vi "CmdCenter_RFmx_Test.vi"(8 "error in (no error)":errorcluster, 11 "Message_Queues":T4) -> (0 "error out":errorcluster)   [LabVIEW 2014]
uses:
  15_DataManagement/Config_RFSG.ctl
  02_Controls/Message_Queues.ctl
  02_Controls/Message_Data_Ctl.ctl
  15_DataManagement/Config_RFmx_Settings.ctl
  15_DataManagement/RFmx_Analysis_Parameter.ctl
panel:
  in  "RFmx_An_Data":T1={"Center_Freq(Hz)"=1000000000.0, "Span(Hz)"=30000000.0, "Ch_IBW(Hz)"=3840000.0, "IMD_Tone_Spacing(Hz)"=3000000.0, "IMD_Span(Hz)"=30000000.0, "IMD_Ch_IBW(Hz)"=1000000.0, "IMD_TargPwr(dBm)"=-10.0, "SFDR_Span(Hz)"=50000000.0, "SFDR_Ch_IBW(Hz)"=2000000.0, "ACP_Offset_Freq"=[10000000.0, 7500000.0, 12500000.0], "ACP_Offset_IBW"=[9000000.0, 3840000.0, 3840000.0], "Display ?"=TRUE} {"ACP_Offset_IBW" format="%#_6p"; "ACP_Offset_Freq" format="%#_6p"; "SFDR_Ch_IBW(Hz)" format="%.3p"; "SFDR_Span(Hz)" format="%.3p"; "IMD_TargPwr(dBm)" format="%.3p"; "IMD_Ch_IBW(Hz)" format="%.3p"; "IMD_Span(Hz)" format="%.3p"; "IMD_Tone_Spacing(Hz)" format="%.3p"; "Ch_IBW(Hz)" format="%.3p"; "Span(Hz)" format="%.3p"; "Center_Freq(Hz)" format="%.3p"}
  in  "DispOn":bool
  in  "Fetch_Types":string[](array[string])=["Spectrum_Disp", "ACP_Data", "CHP_Data", "OBW_Data", "TXP_Data", "TXP_Disp", "CCDF_Data", "CCDF_Disp", "Harmonics_Disp"]
  in  "Meas_Types":string[](array[string])=["Spectrum", "ACP", "CHP", "OBW", "TXP", "CCDF", "Harmonics"]
  in  "RFmx_Parameters":T2={"Default"={"Center_Freq(Hz)"=1000000000.0, "Ref_Level(dBm)"=-5.0, "Span(Hz)"=30000000.0, "RBW(Hz)"=10000.0, "RBW Filter Type"=enum."Gaussian", "Ch_IBW(Hz)"=3840000.0, "Sweep_Time(s)"=0.01, "Num_of_Average"=10, "IQ_Bandwidth(Hz)"=20000000.0}, "ACP_Offset_Freq"=[10000000.0, 7500000.0, 12500000.0], "ACP_Offset_IBW"=[9000000.0, 3840000.0, 3840000.0], "OBW_Percent(%)"=95.0, "TXP_Interval(s)"=0.01, "CCDF_Interval(s)"=0.01, "CCDF_Threshold"=-30.0, "SFDR_Span(Hz)"=20000000.0, "Harms_RBW(Hz)"=100000.0, "Harms_RBW_Filter"=enum."Gaussian"} {"Harms_RBW(Hz)" format="%.3p"; "TXP_Interval(s)" format="%#_6p"; "SFDR_Span(Hz)" format="%#_6p"; "CCDF_Threshold" format="%#_6p"; "CCDF_Interval(s)" format="%#_6p"; "OBW_Percent(%)" format="%#_6p"; "ACP_Offset_IBW" format="%#_6p"; "ACP_Offset_Freq" format="%#_6p"; "Default"."IQ_Bandwidth(Hz)" format="%#_6p"; "Default"."Sweep_Time(s)" format="%#_6p"; "Default"."Ch_IBW(Hz)" format="%.3p"; "Default"."RBW(Hz)" format="%.3p"; "Default"."Span(Hz)" format="%.3p"; "Default"."Ref_Level(dBm)" format="%.3p"; "Default"."Center_Freq(Hz)" format="%.3p"}
  in  "Config_RFSG":T3={"Carrier Frequency"=1000000000.0, "RF Power Level (dBm)"=-10.0, "SG External Gain (dBm)"=0.0, "Standard"=enum."WCDMA"} {"SG External Gain (dBm)" format="%#_6p"; "RF Power Level (dBm)" format="%#_6p"; "Carrier Frequency" format="%#_6p"}
  out "Current_Message":string="OK"
  in  "Stop Button":bool
  in  "Start":bool
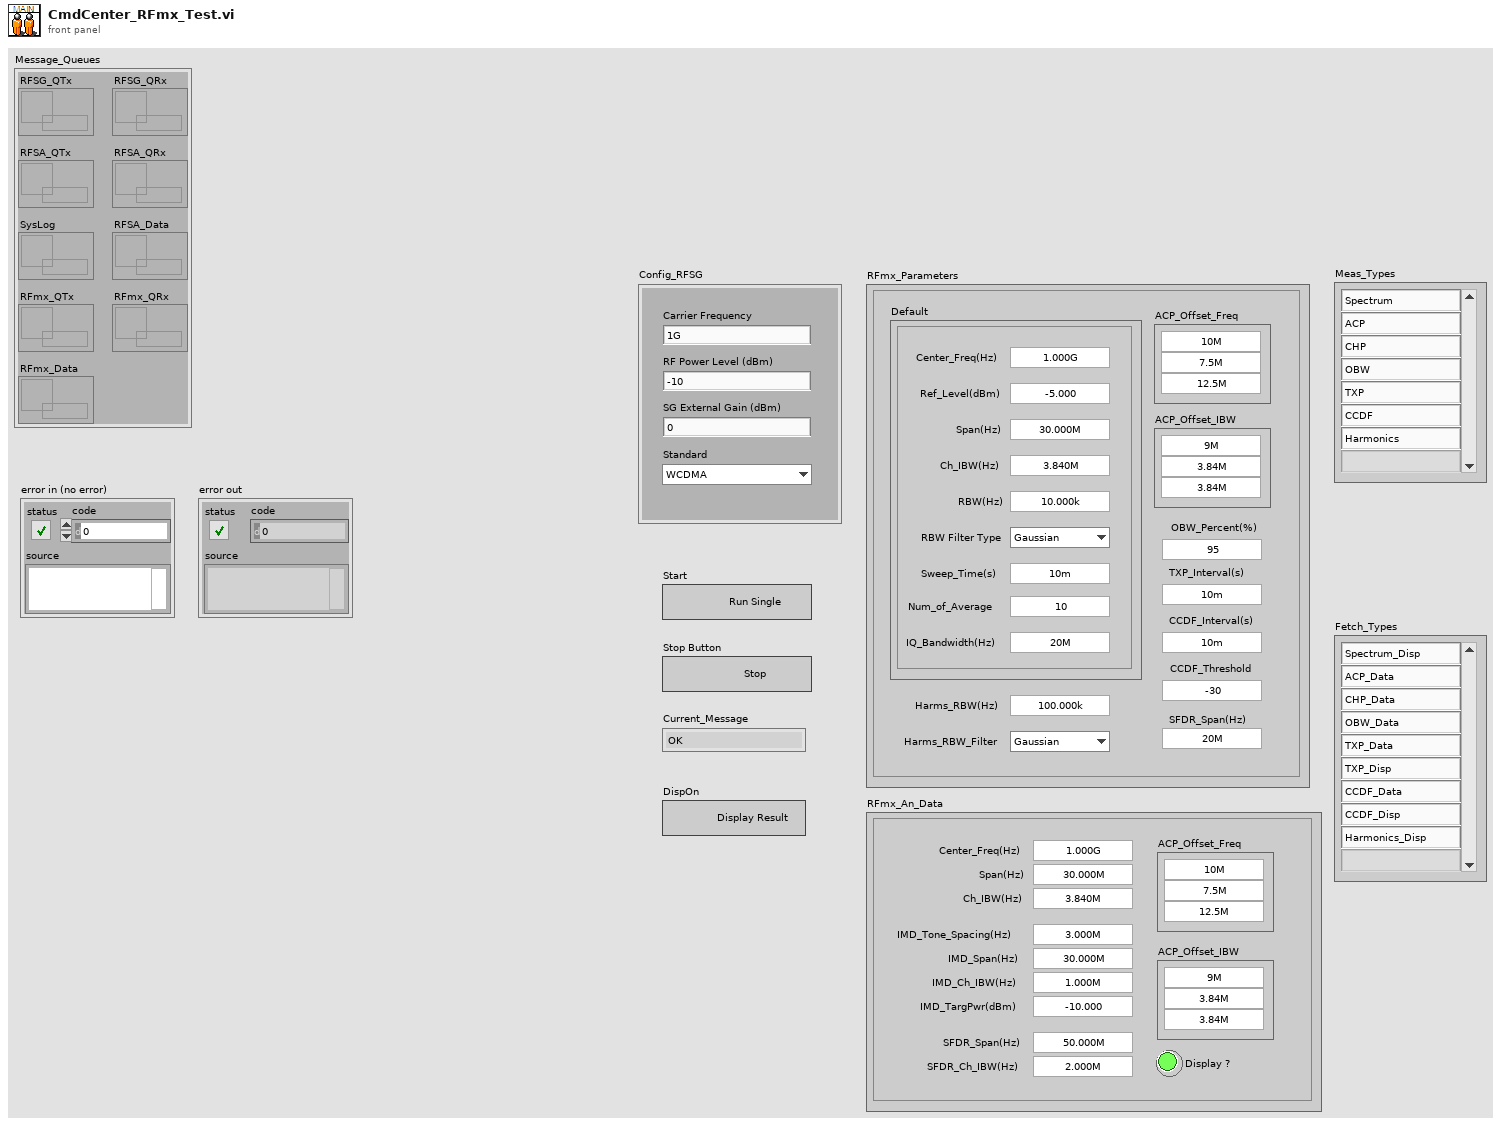
[diagram p1: front panel]
types:
  T1 = typedef "RFmx_Analysis_Parameter.ctl" = cluster{"Center_Freq(Hz)":dbl, "Span(Hz)":dbl, "Ch_IBW(Hz)":dbl, "IMD_Tone_Spacing(Hz)":dbl, "IMD_Span(Hz)":dbl, "IMD_Ch_IBW(Hz)":dbl, "IMD_TargPwr(dBm)":dbl, "SFDR_Span(Hz)":dbl, "SFDR_Ch_IBW(Hz)":dbl, "ACP_Offset_Freq":dbl[], "ACP_Offset_IBW":dbl[], "Display ?":bool}
  T2 = typedef "Config_RFmx_Settings.ctl" = cluster{"Default":cluster{"Center_Freq(Hz)":dbl, "Ref_Level(dBm)":dbl, "Span(Hz)":dbl, "RBW(Hz)":dbl, "RBW Filter Type":enum16{"FFT Based", "Gaussian", "Flat", "Synch Tuned - 4", "Synch Tuned - 5"}, "Ch_IBW(Hz)":dbl, "Sweep_Time(s)":dbl, "Num_of_Average":i32, "IQ_Bandwidth(Hz)":dbl}, "ACP_Offset_Freq":dbl[], "ACP_Offset_IBW":dbl[], "OBW_Percent(%)":dbl, "TXP_Interval(s)":dbl, "CCDF_Interval(s)":dbl, "CCDF_Threshold":dbl, "SFDR_Span(Hz)":dbl, "Harms_RBW(Hz)":dbl, "Harms_RBW_Filter":enum16{"FFT Based", "Gaussian", "Flat", "Synch Tuned - 4", "Synch Tuned - 5"}}
  T3 = typedef "Config_RFSG.ctl" = cluster{"Carrier Frequency":dbl, "RF Power Level (dBm)":dbl, "SG External Gain (dBm)":dbl, "Standard":enum16{"LTE", "WCDMA", "GSM", "EDGE", "CW", "CWM"}}
  T4 = typedef "Message_Queues.ctl" = cluster{"RFSG_QTx":refnum<queue>, "RFSG_QRx":refnum<queue>, "RFSA_QTx":refnum<queue>, "RFSA_QRx":refnum<queue>, "SysLog":refnum<queue>, "RFSA_Data":refnum<queue>, "RFmx_QTx":refnum<queue>, "RFmx_QRx":refnum<queue>, "RFmx_Data":refnum<queue>}
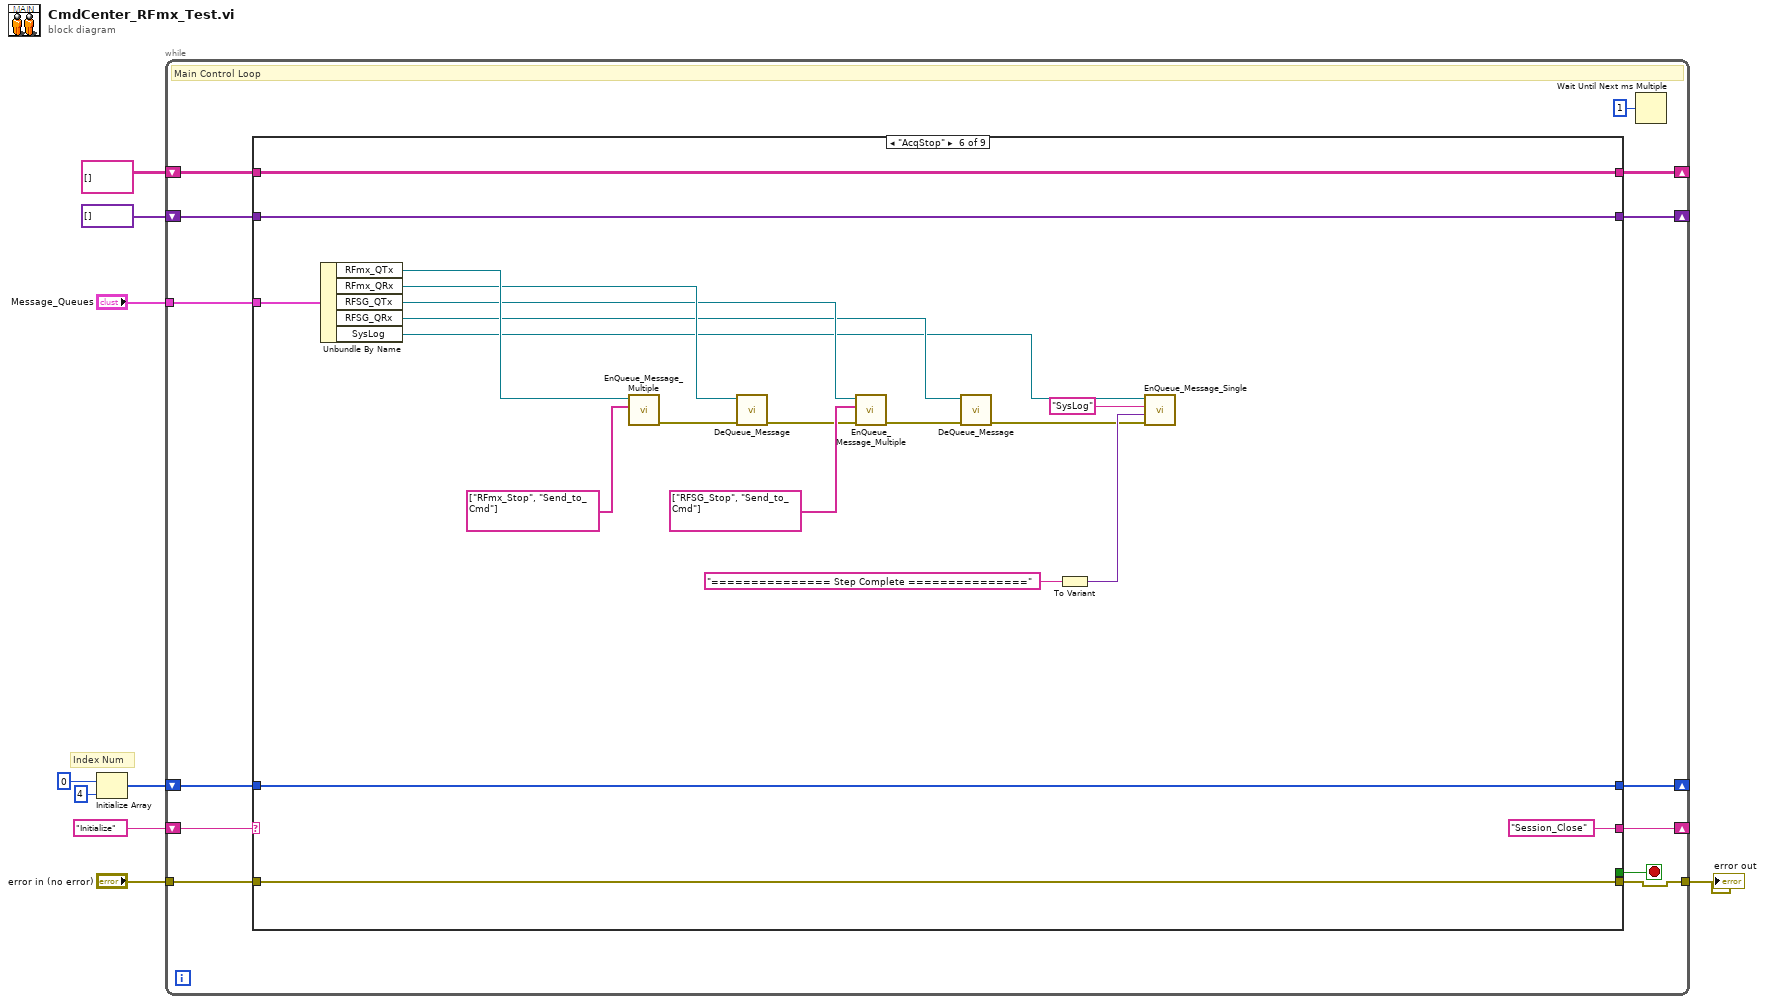
[diagram p0: block diagram]
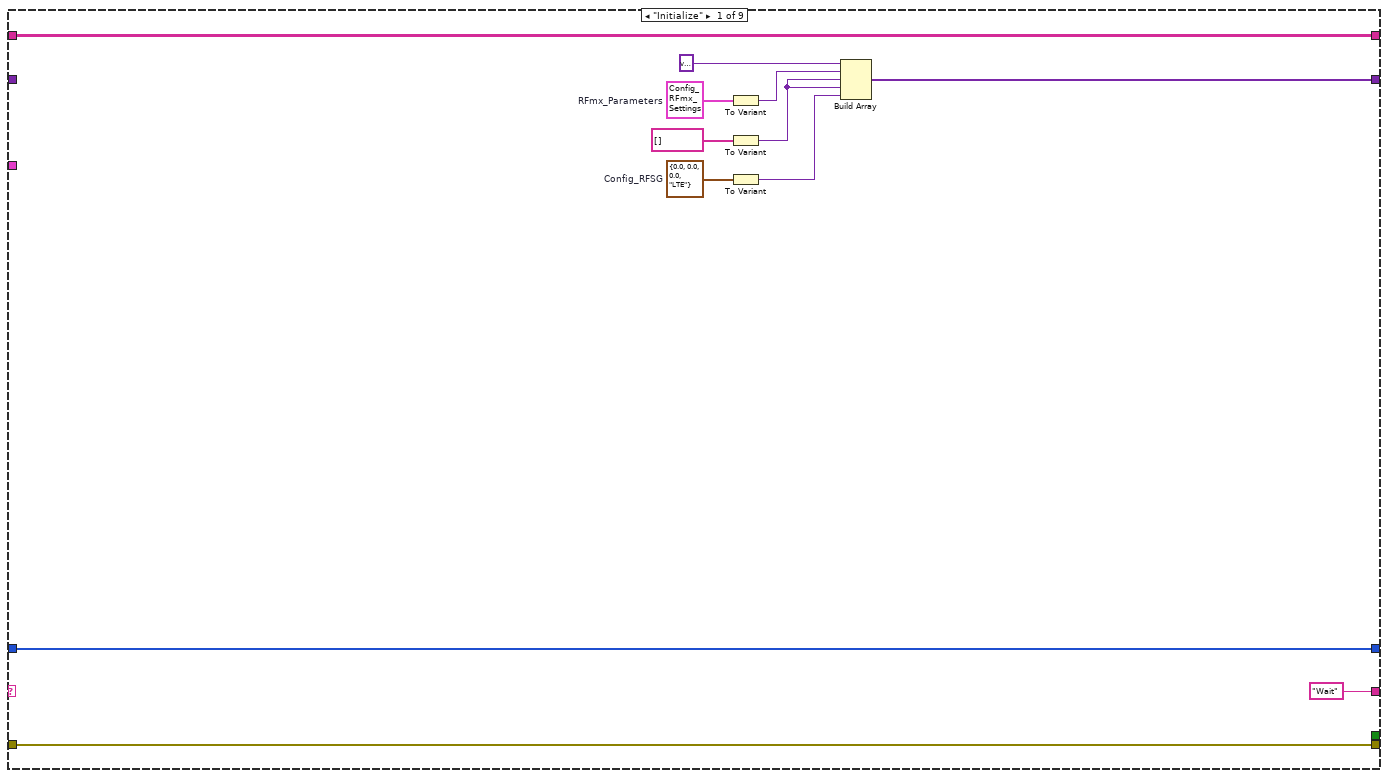
[diagram p2: hidden frame]
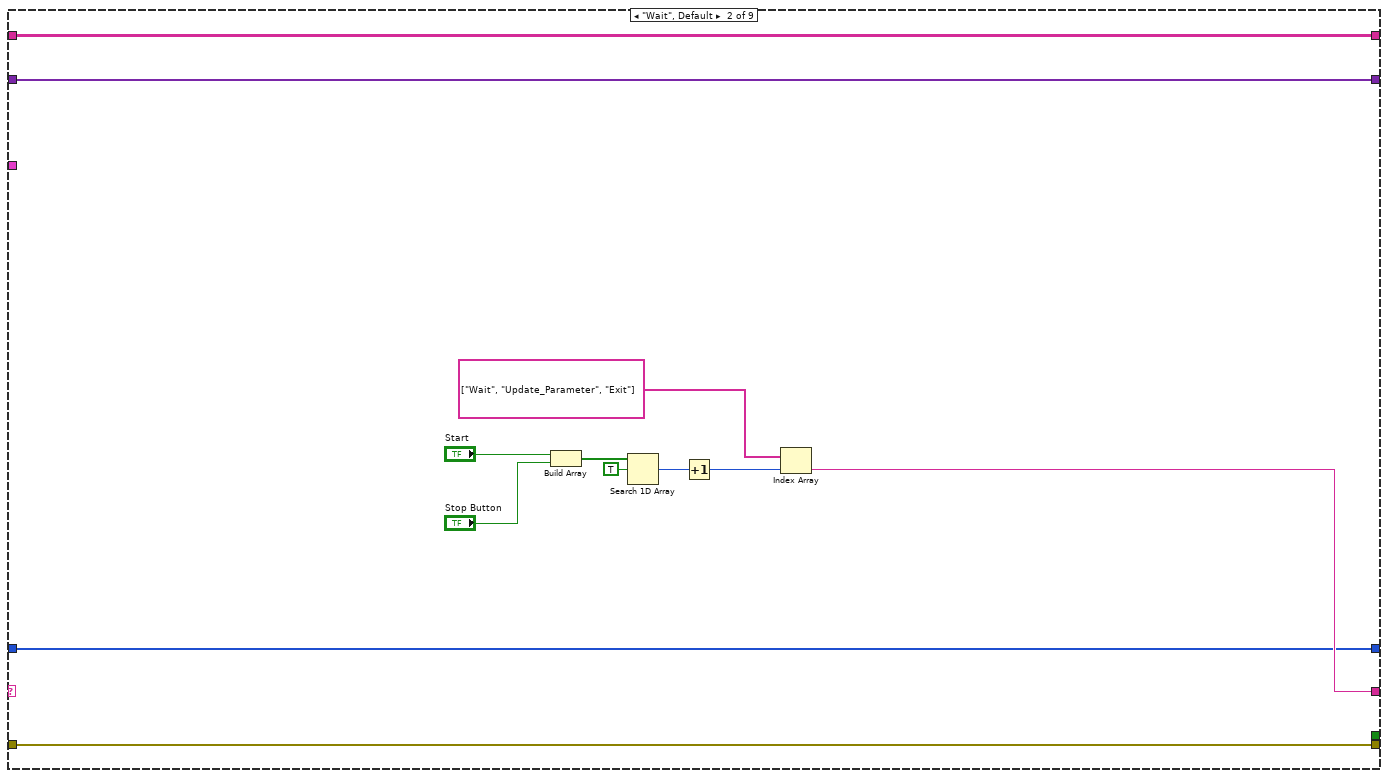
[diagram p3: hidden frame]
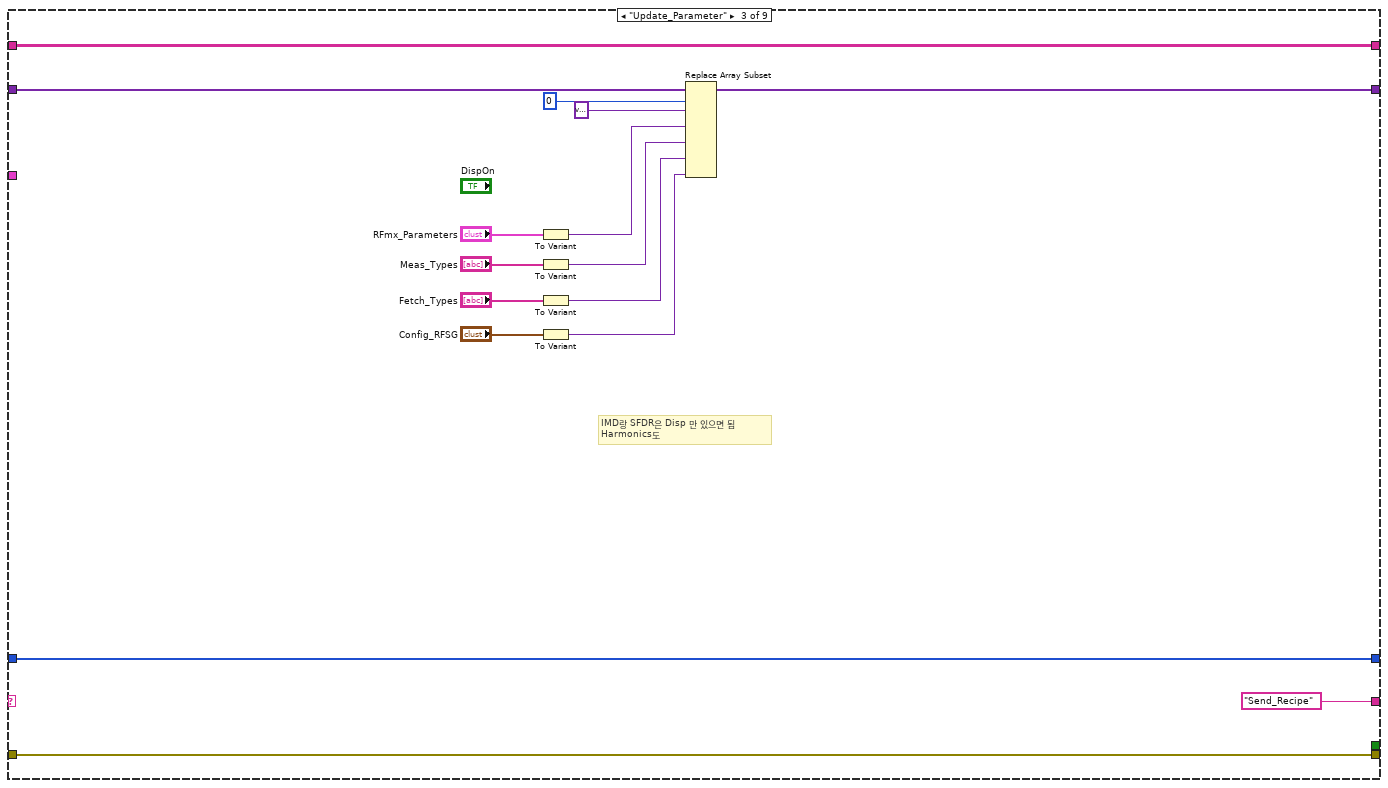
[diagram p4: hidden frame]
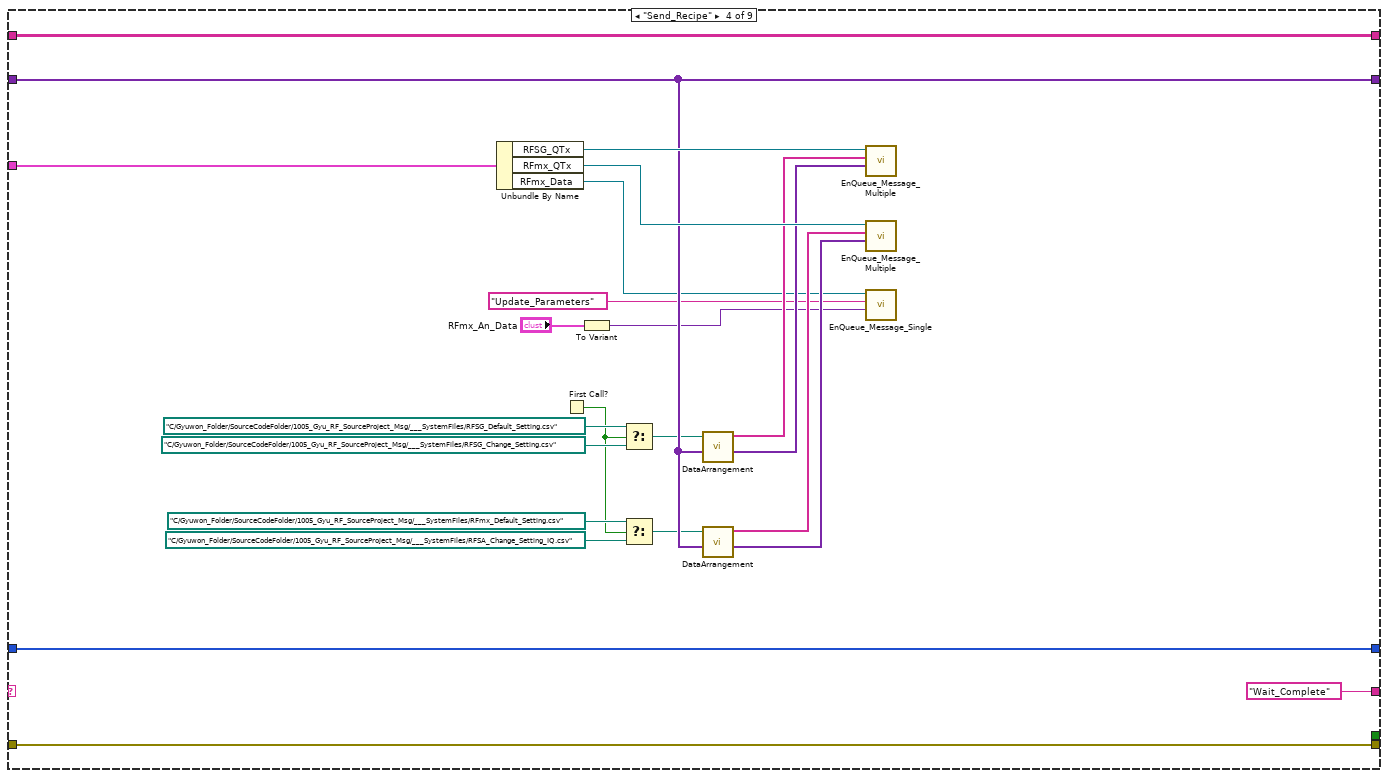
[diagram p5: hidden frame]
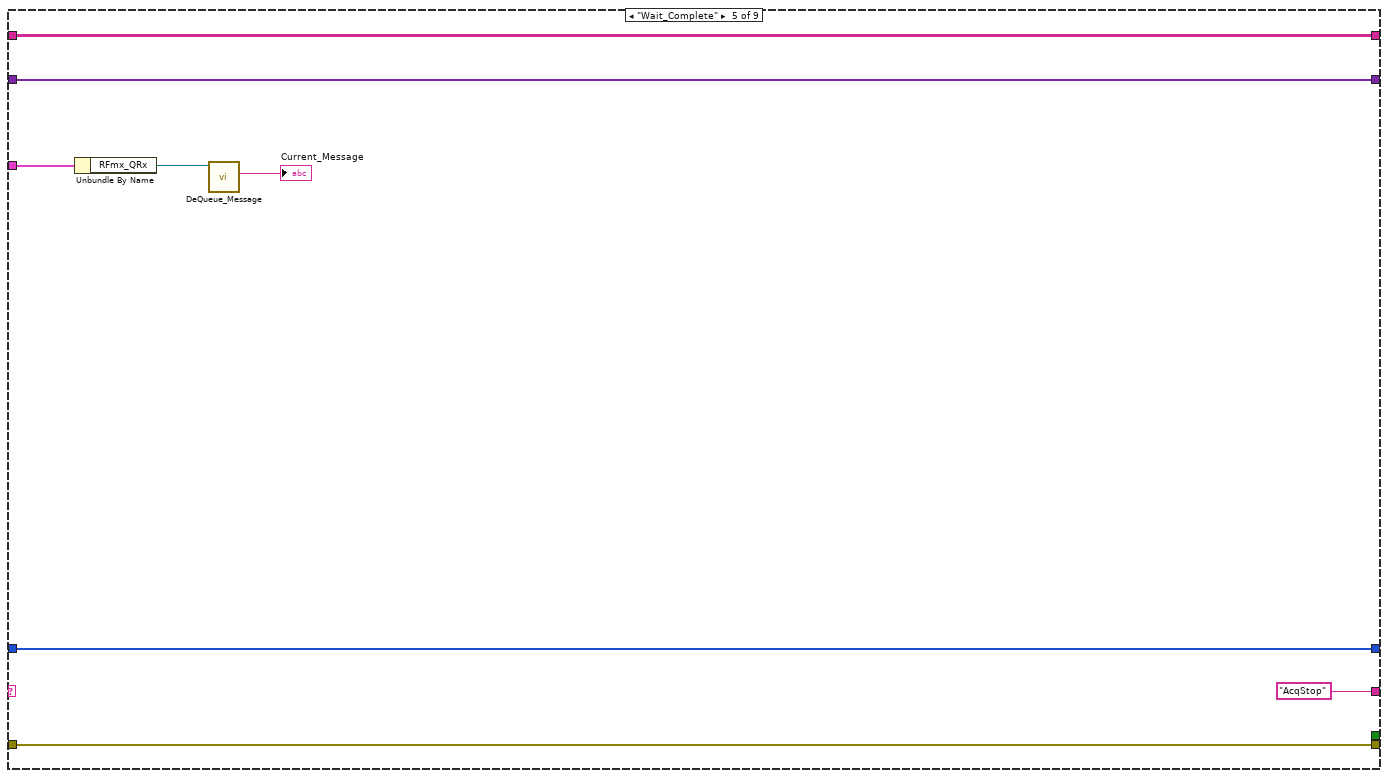
[diagram p6: hidden frame]
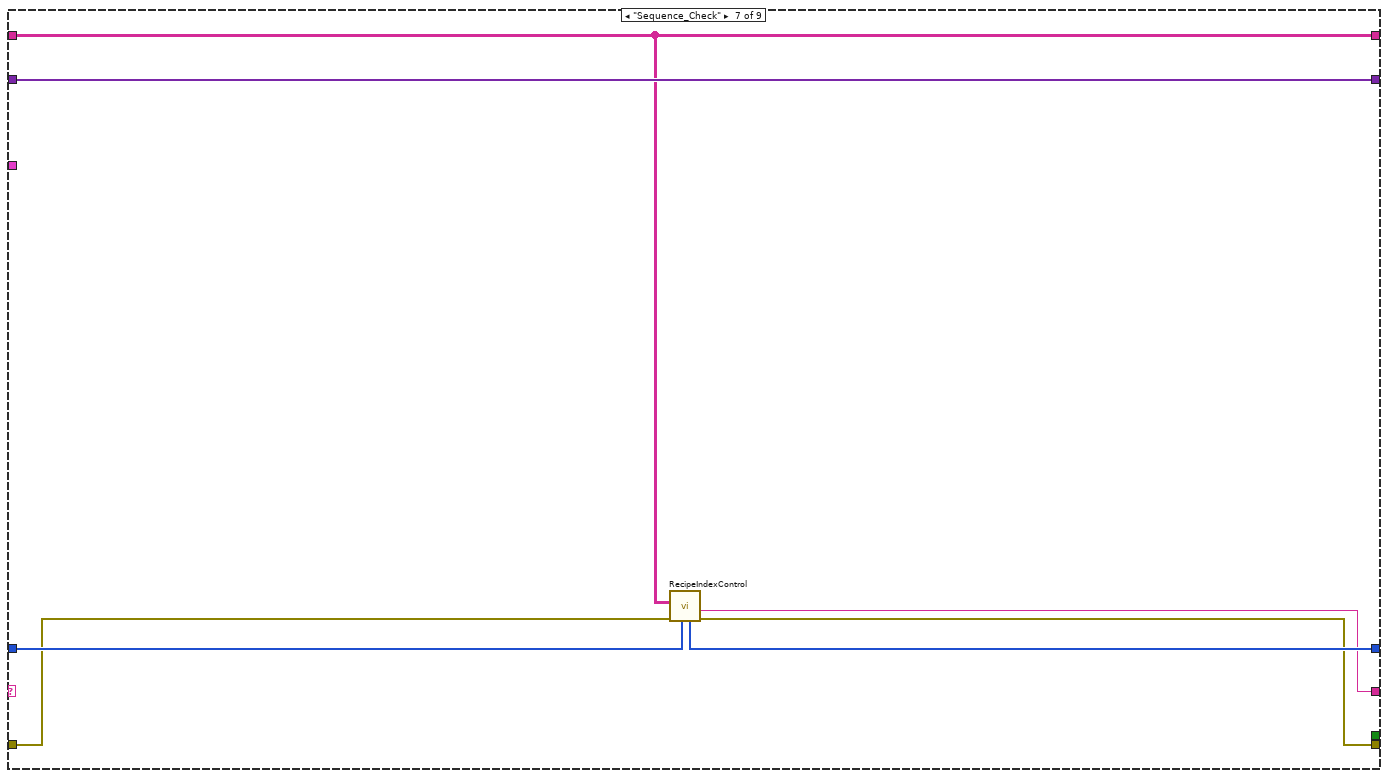
[diagram p7: hidden frame]
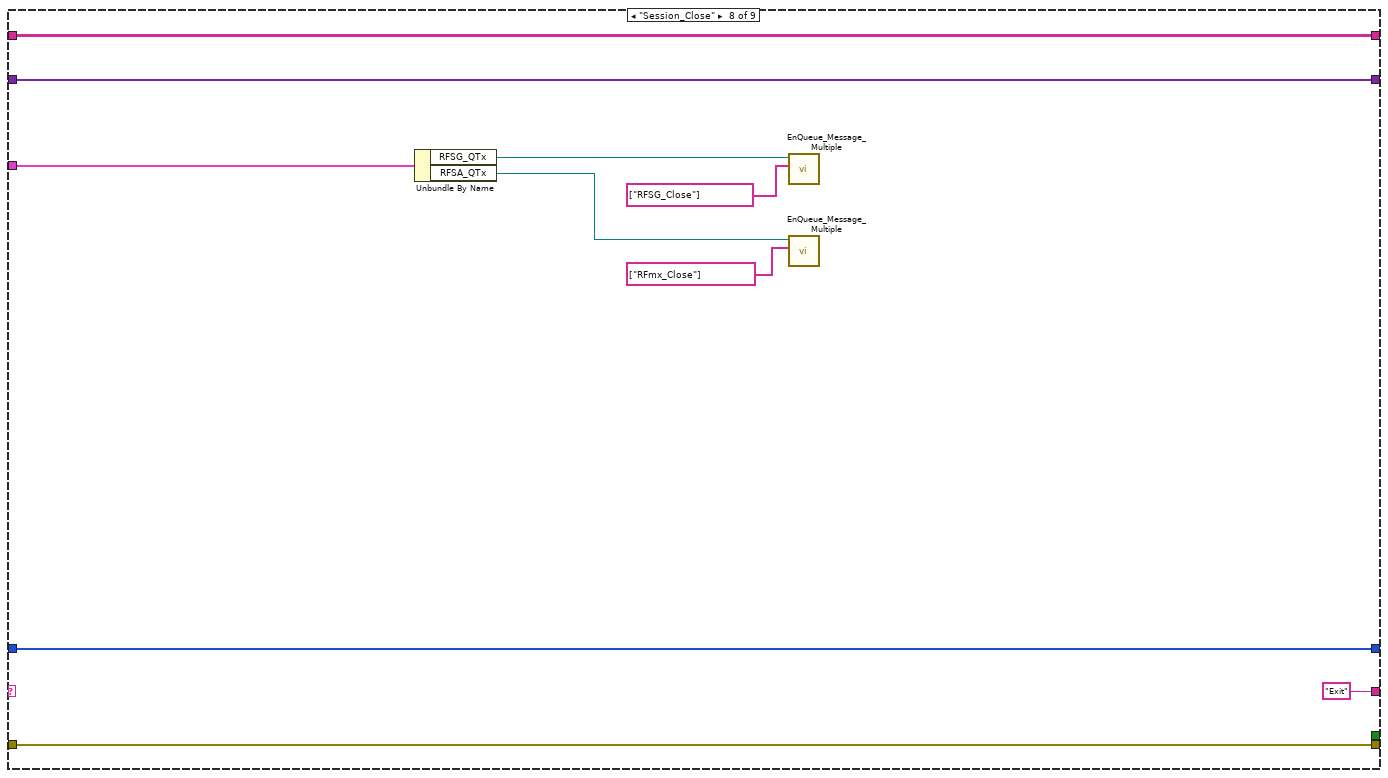
[diagram p8: hidden frame]
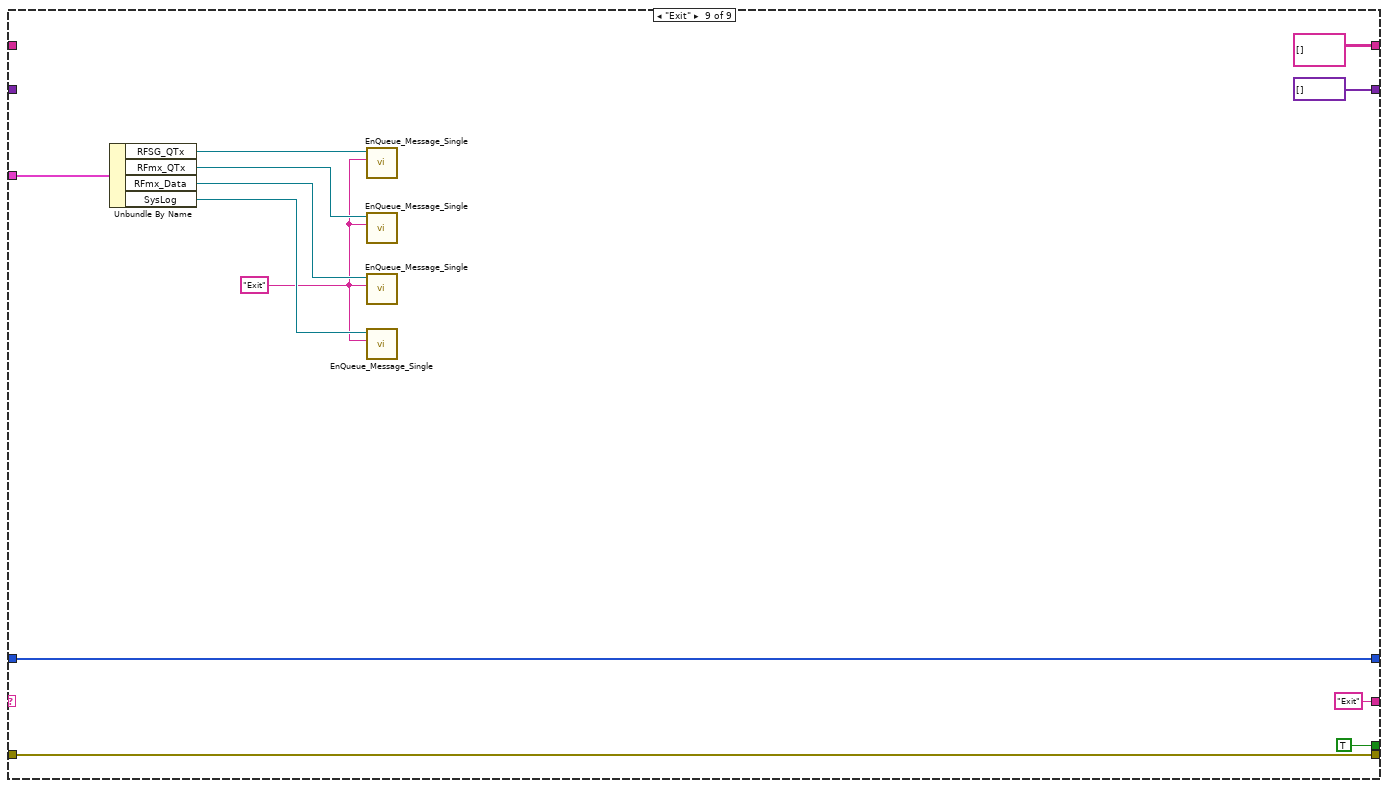
[diagram p9: hidden frame]
diagram:
  # "Index Num"
  n1 = Initialize Array(0, 4 ("dimension size")) -> (w1:i32[])
  n2 = while {
    tunnel: "error in (no error)" -> [w18]
    tunnel: [w21] -> w8
    tunnel: "Message_Queues" -> [w19]
    shift-right: [w16] -> _
    shift-left: "Initialize" -> [w20]
    shift-right: [w14] -> _
    shift-left: variant[] [] ("appended array") -> [w15]
    shift-right: [w13] -> _
    shift-left: string[][] [] ("all rows") -> [w12]
    shift-right: [w10] -> _
    shift-left: w1 -> [w11]
    stop <- w22 stop-if-true
    # "Main Control Loop"
    n3 = case shown="\"AcqStop\"" w20 {
      tunnel: w18 -> [w34 w46 w53 w85 w93 w110 w117 w124 w141]
      tunnel: [_ _ _ _ _ _ _ _ TRUE] -> w22
      tunnel: [w34 w46 w53 w85 w93 w110 w114 w124 w141] -> w21
      tunnel: w19 -> [_ _ _ w84 w91 w112 _ w129 w139]
      tunnel: ["Wait" w40 "Send_Recipe" "Wait_Complete" "AcqStop" "Session_Close" w116 "Exit" "Exit"] -> w16
      tunnel: w15 -> [_ w39 w59 w76 w88 w109 w120 w123 _]
      tunnel: [w31 w39 w58 w76 w88 w109 w120 w123 variant[] [] ("appended array")] -> w14
      tunnel: [w30 w38 w61 w75 w87 w108 w115 w122 string[][] [] ("all rows")] -> w13
      tunnel: w12 -> [w30 w38 w61 w75 w87 w108 w115 w122 _]
      tunnel: w11 -> [w29 w37 w60 w74 w86 w107 w119 w121 w131]
      tunnel: [w29 w37 w60 w74 w86 w107 w118 w121 w131] -> w10
      frame "Initialize" {
        w28 = T2 {"Default"={"Center_Freq(Hz)"=1150000000.0, "Ref_Level(dBm)"=-10.0, "Span(Hz)"=20000000.0, "RBW(Hz)"=10000.0, "RBW Filter Type"=enum."Gaussian", "Ch_IBW(Hz)"=3840000.0, "Sweep_Time(s)"=0.01, "Num_of_Average"=10, "IQ_Bandwidth(Hz)"=20000000.0}, "ACP_Offset_Freq"=[5000000.0, 10000000.0, 12500000.0], "ACP_Offset_IBW"=[3840000.0, 3840000.0, 3840000.0], "OBW_Percent(%)"=95.0, "TXP_Interval(s)"=0.01, "CCDF_Interval(s)"=0.01, "CCDF_Threshold"=-30.0, "SFDR_Span(Hz)"=20000000.0, "Harms_RBW(Hz)"=10000.0, "Harms_RBW_Filter"=enum."Gaussian"}  # RFmx_Parameters
        w32 = T3 {"Carrier Frequency"=0.0, "RF Power Level (dBm)"=0.0, "SG External Gain (dBm)"=0.0, "Standard"=enum."LTE"}  # Config_RFSG
        n4 = To Variant(anything=w28) -> (Variant=w27:variant)
        n5 = To Variant(anything=string[] []) -> (Variant=w23:variant)
        n6 = To Variant(anything=w32) -> (Variant=w26:variant)
        n7 = Build Array(variant ("element"), w27, w23, w23, w26) -> (w31:variant[])
      }
      frame "Wait", Default {
        n8 = Build Array("Start", "Stop Button") -> (w44:bool[])
        n9 = Search 1D Array(1D array=w44, element=TRUE) -> (index of element=w42:i32)  [unwired: 1 in]
        n10 = Increment(x=w42) -> (x+1=w41:i32)
        n11 = Index Array(array=string[] ["Wait", "Update_Parameter", "Exit"], index=w41) -> (element=w40:string)
      }
      frame "Update_Parameter" {
        # "IMD랑 SFDR은 Disp 만 있으면 됨\nHarmonics도"
        n12 = To Variant(anything="RFmx_Parameters") -> (Variant=w54:variant)
        n13 = To Variant(anything="Meas_Types") -> (Variant=w51:variant)
        n14 = To Variant(anything="Fetch_Types") -> (Variant=w47:variant)
        n15 = To Variant(anything="Config_RFSG") -> (Variant=w49:variant)
        n16 = Replace Array Subset(array=w59, new element #1=variant ("new element/subarray"), index #1=0 ("index"), new element #2=w54, new element #3=w51, new element #4=w47, new element #5=w49) -> (w58:variant[])  [unwired: 4 in]
      }
      frame "Send_Recipe" {
        n17 = Unbundle By Name(w84) -> ("RFSG_QTx"=w83:refnum<queue>, "RFmx_QTx"=w82:refnum<queue>, "RFmx_Data"=w66:refnum<queue>)
        n18 = First Call?() -> (First Call?: T/F=w69:bool)
        n19 = To Variant(anything="RFmx_An_Data") -> (Variant=w64:variant)
        n20 = Select(t=path "C:/Gyuwon_Folder/SourceCodeFolder/1005_Gyu_RF_SourceProject_Msg/___SystemFiles/RFSG_Default_Setting.csv" ("RFSG_List_1st"), s=w69, f=path "C:/Gyuwon_Folder/SourceCodeFolder/1005_Gyu_RF_SourceProject_Msg/___SystemFiles/RFSG_Change_Setting.csv" ("RFSG_List_1st")) -> (s? t:f=w68:path)
        n21 = Select(t=path "C:/Gyuwon_Folder/SourceCodeFolder/1005_Gyu_RF_SourceProject_Msg/___SystemFiles/RFmx_Default_Setting.csv" ("RFSA_List_1st"), s=w69, f=path "C:/Gyuwon_Folder/SourceCodeFolder/1005_Gyu_RF_SourceProject_Msg/___SystemFiles/RFSA_Change_Setting_IQ.csv" ("RFSA_List_1st")) -> (s? t:f=w67:path)
        n22 = call "DataArrangement.vi"("DataType"=w76, "file path (dialog if empty)"=w68) -> ("DataList"=w79:variant[], "CmdList"=w80:string[])  [unwired: 7 in, 1 out]
        n23 = call "DataArrangement.vi"("DataType"=w76, "file path (dialog if empty)"=w67) -> ("DataList"=w77:variant[], "CmdList"=w78:string[])  [unwired: 7 in, 1 out]
        n24 = call "EnQueue_Message_Multiple.vi"("Message Data Array"=w79, "Message Array"=w80, "Message_Queue"=w83) -> ()  [unwired: 7 in, 2 out]
        n25 = call "EnQueue_Message_Multiple.vi"("Message Data Array"=w77, "Message Array"=w78, "Message_Queue"=w82) -> ()  [unwired: 7 in, 2 out]
        n26 = call "EnQueue_Message_Single.vi"("Message Data"=w64, "Message"="Update_Parameters", "Message_Queue"=w66) -> ()  [unwired: 7 in, 2 out]
      }
      frame "Wait_Complete" {
        n27 = Unbundle By Name(w91) -> ("RFmx_QRx"=w90:refnum<queue>)
        n28 = call "DeQueue_Message.vi"("Message_Queue"=w90) -> ("Message"=→"Current_Message":string)  [unwired: 7 in, 3 out]
      }
      frame "AcqStop" {
        n29 = Unbundle By Name(w112) -> ("RFmx_QTx"=w106:refnum<queue>, "RFmx_QRx"=w105:refnum<queue>, "RFSG_QTx"=w103:refnum<queue>, "RFSG_QRx"=w101:refnum<queue>, "SysLog"=w100:refnum<queue>)
        n30 = call "EnQueue_Message_Multiple.vi"("Message Array"=string[] ["RFmx_Stop", "Send_to_Cmd"], "Message_Queue"=w106) -> ("error out"=w94:errorcluster)  [unwired: 8 in, 1 out]
        n31 = call "DeQueue_Message.vi"("error in (no error)"=w94, "Message_Queue"=w105) -> ("error out"=w95:errorcluster)  [unwired: 6 in, 3 out]
        n32 = call "EnQueue_Message_Multiple.vi"("error in (no error)"=w95, "Message Array"=string[] ["RFSG_Stop", "Send_to_Cmd"], "Message_Queue"=w103) -> ("error out"=w102:errorcluster)  [unwired: 7 in, 1 out]
        n33 = call "DeQueue_Message.vi"("error in (no error)"=w102, "Message_Queue"=w101) -> ("error out"=w96:errorcluster)  [unwired: 6 in, 3 out]
        n34 = To Variant(anything="=============== Step Complete ===============" ("Message")) -> (Variant=w97:variant)
        n35 = call "EnQueue_Message_Single.vi"("error in (no error)"=w96, "Message Data"=w97, "Message"="SysLog", "Message_Queue"=w100) -> ()  [unwired: 6 in, 2 out]
      }
      frame "Sequence_Check" {
        n36 = call "RecipeIndexControl.vi"("Index_List"=w119, "error in (no error)"=w117, "Recipe_Input"=w115) -> ("error out"=w114:errorcluster, "Status"=w116:string, "Index_List_out"=w118:i32[])  [unwired: 6 in]
      }
      frame "Session_Close" {
        n37 = Unbundle By Name(w129) -> ("RFSG_QTx"=w128:refnum<queue>, "RFSA_QTx"=w126:refnum<queue>)
        n38 = call "EnQueue_Message_Multiple.vi"("Message Array"=string[] ["RFSG_Close"], "Message_Queue"=w128) -> ()  [unwired: 8 in, 2 out]
        n39 = call "EnQueue_Message_Multiple.vi"("Message Array"=string[] ["RFmx_Close"], "Message_Queue"=w126) -> ()  [unwired: 8 in, 2 out]
      }
      frame "Exit" {
        w134 = "Exit" ("Message")
        n40 = Unbundle By Name(w139) -> ("RFSG_QTx"=w138:refnum<queue>, "RFmx_QTx"=w137:refnum<queue>, "RFmx_Data"=w136:refnum<queue>, "SysLog"=w135:refnum<queue>)
        n41 = call "EnQueue_Message_Single.vi"("Message"=w134, "Message_Queue"=w138) -> ()  [unwired: 8 in, 2 out]
        n42 = call "EnQueue_Message_Single.vi"("Message"=w134, "Message_Queue"=w137) -> ()  [unwired: 8 in, 2 out]
        n43 = call "EnQueue_Message_Single.vi"("Message"=w134, "Message_Queue"=w136) -> ()  [unwired: 8 in, 2 out]
        n44 = call "EnQueue_Message_Single.vi"("Message"=w134, "Message_Queue"=w135) -> ()  [unwired: 8 in, 2 out]
      }
    }
    n45 = Wait Until Next ms Multiple(millisecond multiple=u32 1) -> ()  [unwired: 1 out]
  }
  "error out" <- w8
